vi "Drop-offFunc.vi"() -> ()   [LabVIEW 2016, in "Team234_Project5.lvrbt"]
uses:
  Team234_Project5.lvrbt
  <vilib>/NXT/Block Support/NXT_InputPort.ctl
  <vilib>/NXT/Subs/LVHSConnector.ctl
  <vilib>/NXT/LegoClasses/BrickReference/BrickReference.lvclass
  <vilib>/NXT/Block Support/NXT_OutputPort.ctl
  <vilib>/NXT/Dual Mode Library/Sensors/EV3_Ultrasonic_IN.vi
  <vilib>/NXT/NXTIO Xnodes/NXTIONodeSubVIs/NXTMoveMotors.vi
  <vilib>/NXT/Dual Mode Library/Waits/Wait_Num.vi
  <vilib>/NXT/NXTIO Xnodes/AddressXNode/NXTIOAddress.xnode
  <vilib>/NXT/NXTIO Xnodes/NXTIOXNode/NXTIO.xnode
panel:
  out "NXT/EV3 3":T1
  out "NXT/EV3 2":T1
  in  "Time (1 sec)":sgl=1.0
  in  "Power/Speed 1":i8=75
  out "Inches (Output)":sgl
  in  "NXT/EV3":T1
  in  "Ultrasonic Sensor Port\n (Port 3)":T2 items=["Port 1", "Port 2", "Port 3", "Port 4"]
  # "Timer"
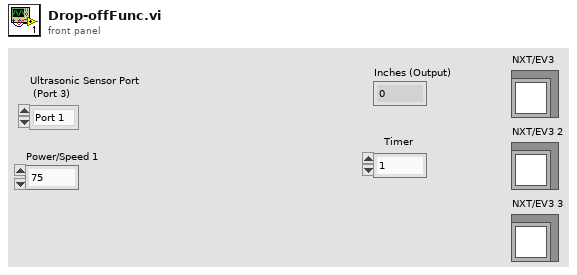
[diagram p1: front panel]
types:
  T1 = typedef "LVHSConnector.ctl" = refnum<class "BrickReference.lvclass">
  T2 = typedef "NXT_InputPort.ctl" = u32
  T3 = typedef "NXT_OutputPort.ctl" = u8
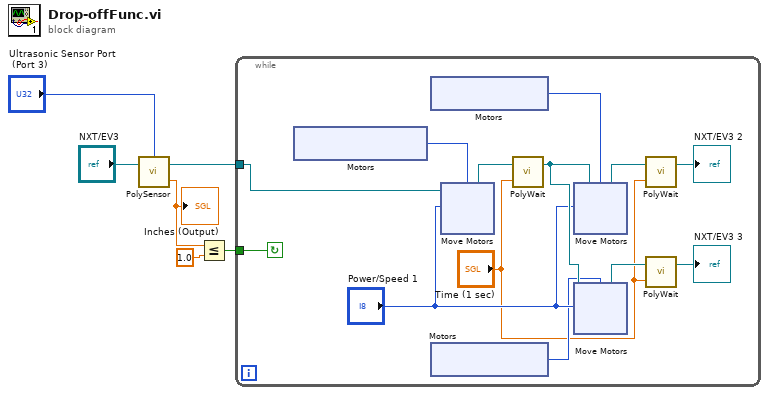
[diagram p0: block diagram]
diagram:
  n1 = call-poly <vilib>:"PolySensor.vi"("NXT/EV3"="NXT/EV3", "Port (Port 1)"="Ultrasonic Sensor Port\n (Port 3)") -> ("Inches"=w3:sgl, "NXT/EV3"=w1:T1)  [unwired: 1 in]
  "Inches (Output)" <- w3
  n2 = Less Or Equal?(x=w3, y=sgl 1.0) -> (x <= y?=w4:bool)
  n3 = while {
    tunnel: w4 -> [w19]
    tunnel: w1 -> [w18]
    stop <- w19 continue-if-true
    n4 = xnode "Motors"() -> ("Motor"=w17:T3)
    n5 = xnode "Motors"() -> ("Motor"=w12:T3)
    n6 = xnode "Motors"() -> ("Motor"=w13:T3)
    n7 = xnode "Move Motors"("Power/Speed 1"="Power/Speed 1", "Motors"=w17, "NXT/EV3"=w18) -> ("NXT/EV3"=w16:T1)
    n8 = call-poly <vilib>:"PolyWait.vi"("Time (1 sec)"="Time (1 sec)", "NXT/EV3"=w16) -> ("NXT/EV3"=w15:T1)  [unwired: 2 in]
    n9 = xnode "Move Motors"("Power/Speed 1"="Power/Speed 1", "Motors"=w12, "NXT/EV3"=w15) -> ("NXT/EV3"=w11:T1)
    n10 = xnode "Move Motors"("Power/Speed 1"="Power/Speed 1", "Motors"=w13, "NXT/EV3"=w15) -> ("NXT/EV3"=w10:T1)
    n11 = call-poly <vilib>:"PolyWait.vi"("Time (1 sec)"="Time (1 sec)", "NXT/EV3"=w11) -> ("NXT/EV3"=→"NXT/EV3 2":T1)  [unwired: 2 in]
    n12 = call-poly <vilib>:"PolyWait.vi"("Time (1 sec)"="Time (1 sec)", "NXT/EV3"=w10) -> ("NXT/EV3"=→"NXT/EV3 3":T1)  [unwired: 2 in]
  }
